vi "TurnToDegrees.vi"(10 "Angle":dbl, 11 "RobotDriveDevRef":T1={"DevStatus"={"status"=FALSE, "code"=0, "source"=""}, "Motors[]"=[], "Square Inputs"=FALSE, "Max Output"=1.0}) -> (3 "RobotDriveDevRef 2":T1={"DevStatus"={"status"=FALSE, "code"=0, "source"=""}, "Motors[]"=[], "Square Inputs"=FALSE, "Max Output"=1.0})   [LabVIEW 2016]
uses:
  <vilib>/Rock Robotics/WPI/RobotDrive/WPI_RobotDriveDevRef.ctl
  <vilib>/Rock Robotics/WPI/MotorControl/WPI_MotorControlDeviceRef.ctl
  <vilib>/Rock Robotics/WPI/MotorControl/WPI_MotorControlType.ctl
  <vilib>/Rock Robotics/SystemInterfaces/DIO/FPGA_DIOPWMChannel.ctl
  <vilib>/Rock Robotics/WPI/PWM/WPI_PWMDeadband.ctl
  Robot Global Data.vi
  <vilib>/addons/control/pid/pid.llb/PID (DBL).vi
  <vilib>/Rock Robotics/WPI/RobotDrive/WPI_RobotDriveArcadeDrive_Standard(NoSaturation).vi
  <vilib>/addons/control/pid/NI_PID_pid.lvlib
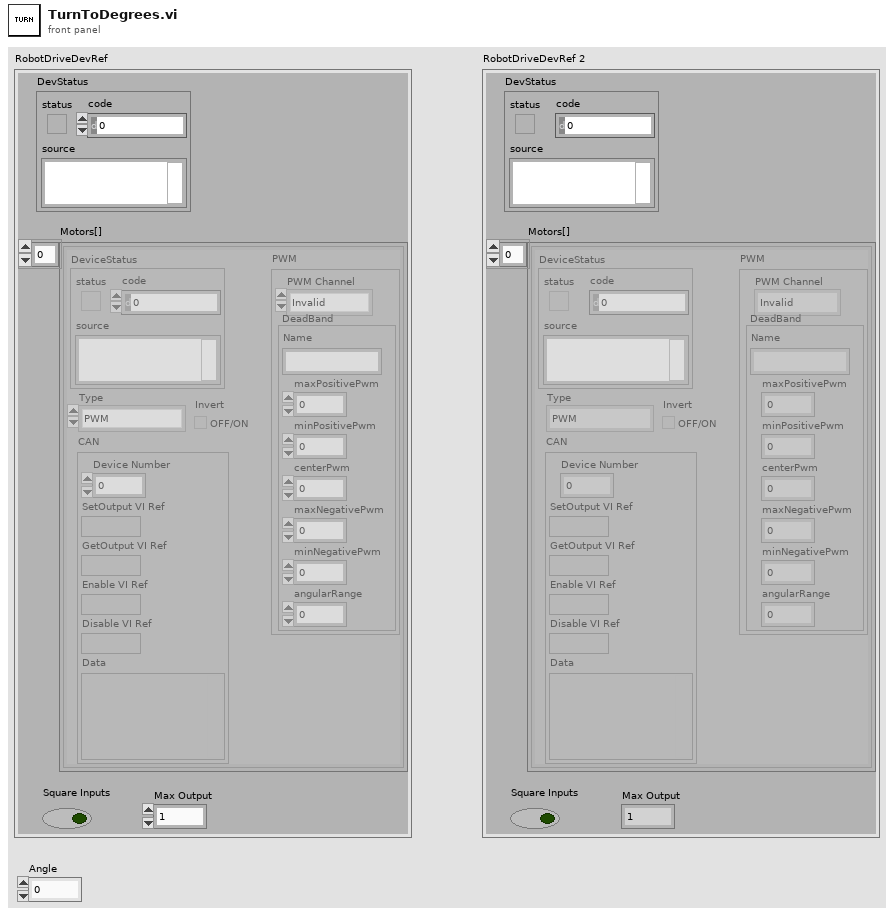
[diagram p1: front panel]
types:
  T1 = typedef "WPI_RobotDriveDevRef.ctl" = cluster{"DevStatus":errorcluster, "Motors[]":T2[], "Square Inputs":bool, "Max Output":dbl}
  T2 = typedef "WPI_MotorControlDeviceRef.ctl" = cluster{"DeviceStatus":errorcluster, "Type":T3, "PWM":cluster{"PWM Channel":T4, "DeadBand":T5}, "CAN":cluster{"Device Number":u8, "SetOutput VI Ref":variant, "GetOutput VI Ref":variant, "Enable VI Ref":variant, "Disable VI Ref":variant, "Data":variant}, "Invert":bool}
  T3 = typedef "WPI_MotorControlType.ctl" = enum16{"PWM", "CAN"}
  T4 = typedef "FPGA_DIOPWMChannel.ctl" = enum8{"PWM 0", "PWM 1", "PWM 2", "PWM 3", "PWM 4", "PWM 5", "PWM 6", "PWM 7", "PWM 8", "PWM 9", "PWM MXP 0", "PWM MXP 1", "PWM MXP 2", "PWM MXP 3", "PWM MXP 4", "PWM MXP 5", "PWM MXP 6", "PWM MXP 7", "PWM MXP 8", "PWM MXP 9", "Invalid"}
  T5 = typedef "WPI_PWMDeadband.ctl" = cluster{"Name":string, "maxPositivePwm":i32, "minPositivePwm":i32, "centerPwm":i32, "maxNegativePwm":i32, "minNegativePwm":i32, "angularRange":u16}
  T6 = cluster{"proportional gain (Kc)":dbl, "integral time (Ti, min)":dbl, "derivative time (Td, min)":dbl}
  T7 = cluster{"proportional gain (Kc)":dbl, "f":dbl, "derivative time (Td, min)":dbl}
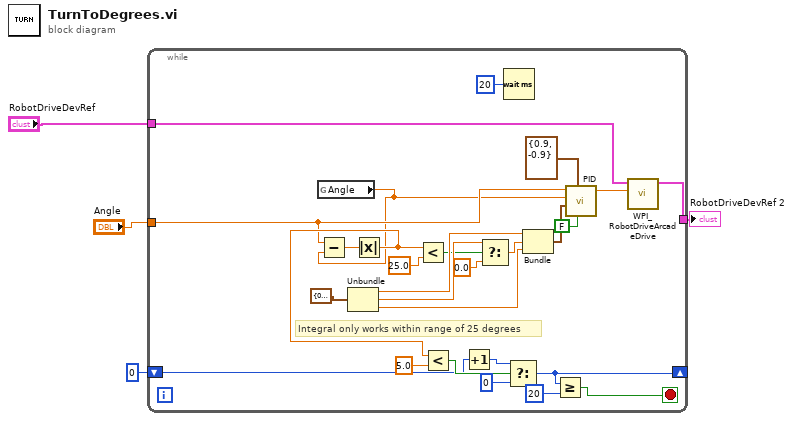
[diagram p0: block diagram]
diagram:
  n1 = while {
    tunnel: "RobotDriveDevRef" -> [w20]
    tunnel: "Angle" -> [w15]
    tunnel: [w16] -> w2
    shift-right: [w8] -> _
    shift-left: 0 -> [w10]
    stop <- w5 stop-if-true
    # "Integral only works within range of 25 degrees"
    n2 = global read "Robot Global Data.vi" "Angle"() -> (w13:dbl)
    n3 = Subtract(x=w15, y=w13) -> (x-y=w29:dbl)
    n4 = Unbundle(T6 {"proportional gain (Kc)"=0.04, "integral time (Ti, min)"=0.005, "derivative time (Td, min)"=0.0018} ("Angle Gains 2")) -> ("proportional gain (Kc)"=w28:dbl, "integral time (Ti, min)"=w26:dbl, "derivative time (Td, min)"=w27:dbl)
    n5 = Absolute Value(x=w29) -> (abs(x)=w18:dbl)
    n6 = Less?(x=w18, y=25.0) -> (x < y?=w25:bool)
    n7 = Less?(x=w18, y=5.0) -> (x < y?=w12:bool)
    n8 = Increment(x=w10) -> (x+1=w11:i32)
    n9 = Select(t=w26, s=w25, f=0.0) -> (s? t:f=w23:dbl)
    n10 = Wait (ms)(milliseconds to wait=u32 20) -> ()  [unwired: 1 out]
    n11 = Select(t=w11, s=w12, f=0) -> (s? t:f=w8:i32)
    n12 = Bundle("proportional gain (Kc)"=w28, "f"=w23, "derivative time (Td, min)"=w27) -> (w22:T7)  [unwired: 1 in]
    n13 = Greater Or Equal?(x=w8, y=20) -> (x >= y?=w5:bool)
    n14 = call-poly <vilib>:"PID.vi"("reinitialize? (F)"=FALSE, "output range"=cluster{"output high":dbl, "output low":dbl} {"output high"=0.9, "output low"=-0.9}, "PID gains"=w22, "process variable"=w13, "setpoint"=w15) -> ("output"=w19:dbl)  [unwired: 5 in, 1 out]
    n15 = call-poly <vilib>:"WPI_RobotDriveArcadeDrive.vi"("X axis value"=w19, "RobotDriveDevRef"=w20) -> ("RobotDriveDevRef"=w16:T1)  [unwired: 7 in, 2 out]
  }
  "RobotDriveDevRef 2" <- w2
